vi "Initialize All DI Channels and TaskRefs.vi"(0 "DAQ":refnum<class "DAQ.lvclass">, 3 "DI Settings[]":T1[](array[typedef]), 5 "DAQNode Dict":T2, 7 "DI Tasks":T3[](array[typedef]), 11 "error in":errorcluster, 14 "Simulate":bool) -> (4 "DAQ out":refnum<class "DAQ.lvclass">, 6 "DAQNode Dict out":T2, 8 "DAQmxTaskDI[]":refnum<k21>[](array[refnum]), 10 "DI TaskNames":string[](array[string]), 15 "error out":errorcluster)   [LabVIEW 2017, in "DAQ.lvclass"]
doc: "Developed by Kevin Thompson\nkevin@thompsonengineering.net\n\nCopyright 2015\nThompson Engineering, LLC"
uses:
  DAQ.lvclass
  DataTypes/TD DI Task--cluster.ctl
  DataTypes/TD DI Channel--cluster.ctl
  <vilib>/TELLC/Dynamic CVT API/TD Dynamic CVT DVR--ref.ctl
  DataTypes/TD DI Instrument Settings--cluster.ctl
  DAQ.lvclass/DAQ.ctl
  Accessors/Set DI IONames.vi
  Accessors/Set DI SchemNames.vi
  Accessors/Set DI Settings.vi
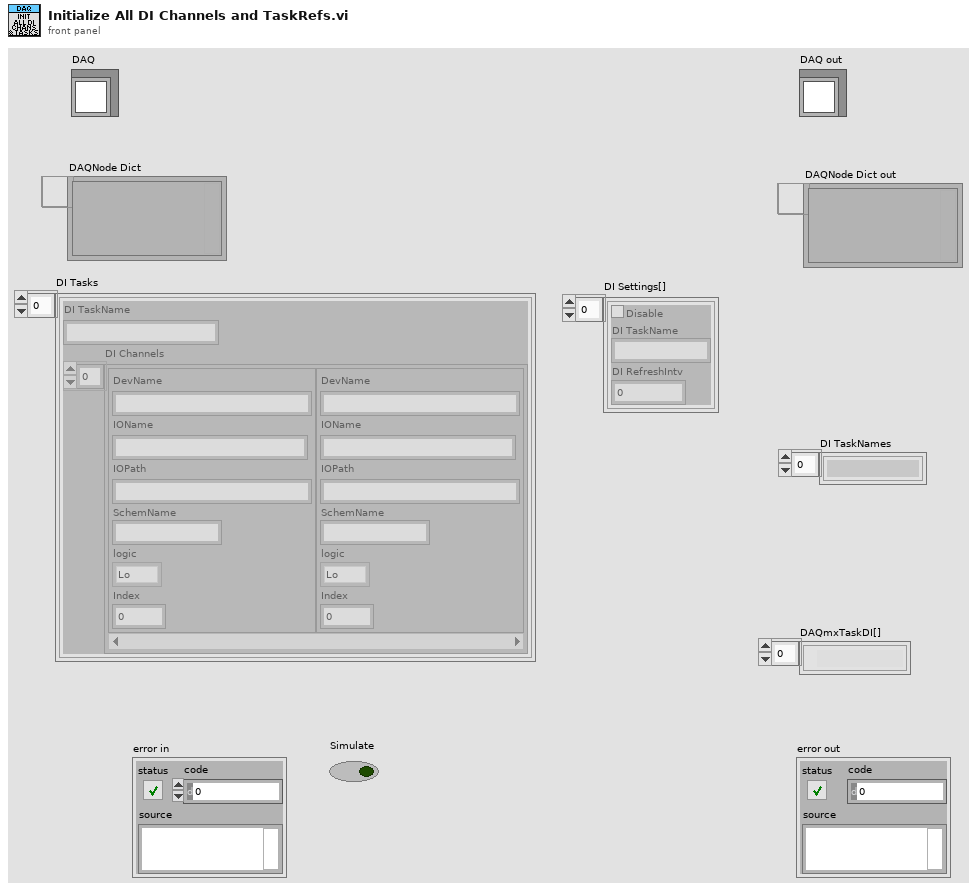
[diagram p1: front panel]
types:
  T1 = typedef "DAQ.lvclass/TD DI Instrument Settings--cluster.ctl" = cluster{"Disable":bool, "DI TaskName":string, "DI RefreshIntv":i32}
  T2 = typedef "TD Dynamic CVT DVR--ref.ctl" = refnum<data-value>
  T3 = typedef "DAQ.lvclass/TD DI Task--cluster.ctl" = cluster{"DI TaskName":string, "DI Channels":T4[]}
  T4 = typedef "DAQ.lvclass/TD DI Channel--cluster.ctl" = cluster{"DevName":string, "IOName":string, "IOPath":string, "SchemName":string, "logic":enum16{"Lo", "Hi"}, "Index":i32}
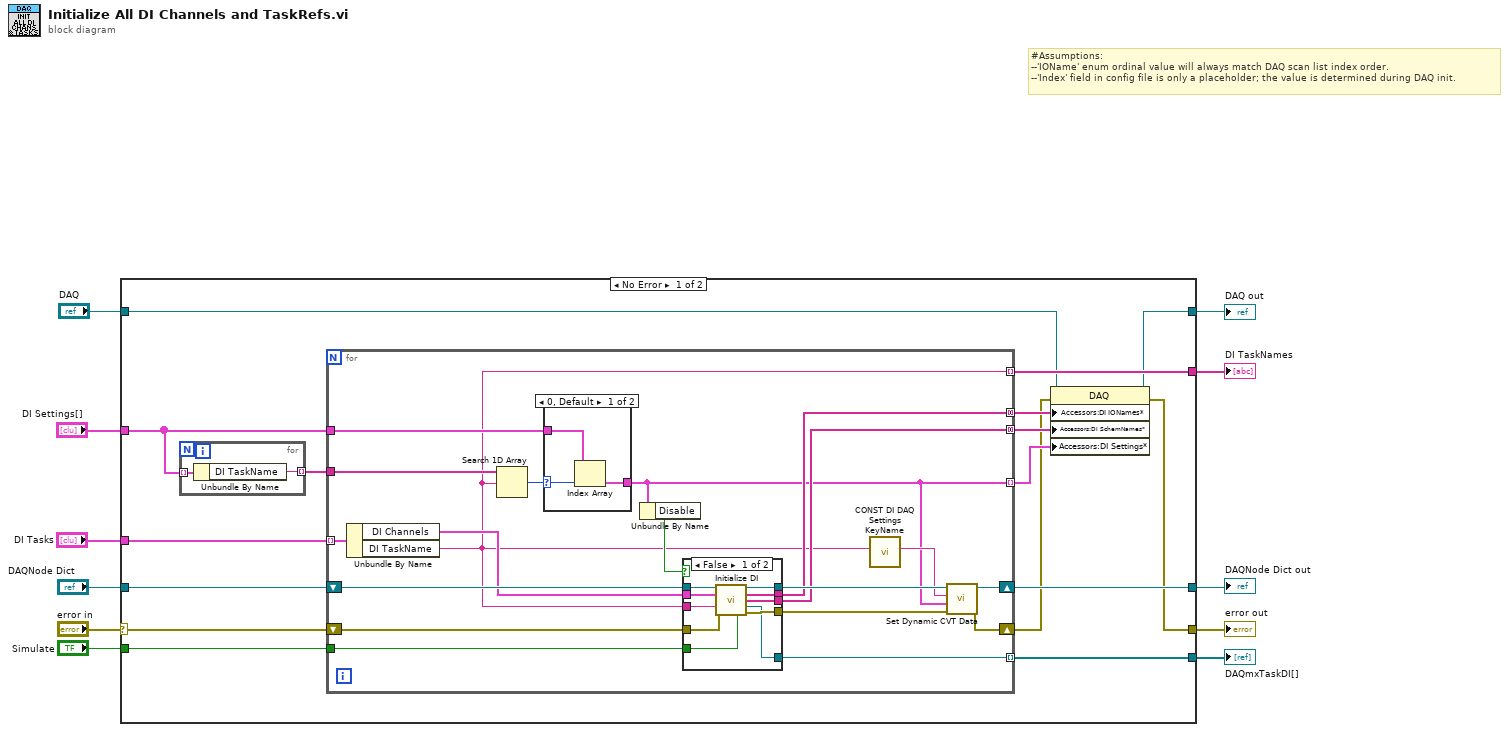
[diagram p0: block diagram]
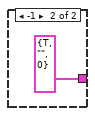
[diagram p3: hidden frame]
diagram:
  # "#Assumptions:\n--'IOName' enum ordinal value will always match DAQ scan list index order.\n--'Index' field in config file is only a placeholder; the value is determined during DAQ init."
  n1 = case shown="No Error" "error in" {
    selector: "error in" -> [w25 w67]
    tunnel: "DI Tasks" -> [w22 _]
    tunnel: "DAQNode Dict" -> [w27 w66]
    tunnel: [w12 w67] -> w9
    tunnel: [w24 w66] -> w4
    tunnel: "Simulate" -> [w26 _]
    tunnel: [w23 _] -> w6
    tunnel: "DI Settings[]" -> [w20 _]
    tunnel: [w19 _] -> w3
    tunnel: [w15 w65] -> w1
    tunnel: "DAQ" -> [w16 w65]
    frame No Error {
      n2 = for {
        tunnel: [w64] -> w21 mode=indexing
        tunnel: w20 -> [w63] mode=indexing
        n3 = Unbundle By Name(w63) -> ("DI TaskName"=w64:string)
      }
      n4 = for {
        tunnel: w26 -> [w34]
        tunnel: [w40] -> w23 mode=indexing
        shift-right: [w43] -> w24
        shift-left: w27 -> [w46]
        shift-right: [w44] -> w13
        shift-left: w25 -> [w45]
        tunnel: w22 -> [w39] mode=indexing
        tunnel: w21 -> [w37]
        tunnel: w20 -> [w35]
        tunnel: [w31] -> w18 mode=concatenating
        tunnel: [w30] -> w17 mode=concatenating
        tunnel: [w29] -> w19 mode=indexing
        tunnel: [w28] -> w14 mode=indexing
        n5 = Unbundle By Name(w39) -> ("DI Channels"=w38:T4[], "DI TaskName"=w29:string)
        n6 = Search 1D Array(1D array=w37, element=w29) -> (index of element=w36:i32)  [unwired: 1 in]
        n7 = case shown="0, Default" w36 {
          selector: w36 -> [w60 _]
          tunnel: [w61 T1 {"Disable"=TRUE, "DI TaskName"="", "DI RefreshIntv"=0} ("DI Settings")] -> w28
          tunnel: w35 -> [w59 _]
          frame 0, Default {
            n8 = Index Array(array=w59, index=w60) -> (element=w61:T1)
          }
          frame -1 {
          }
        }
        n9 = Unbundle By Name(w28) -> ("Disable"=w33:bool)
        n10 = case shown="False" w33 {
          tunnel: w46 -> [w56 w58]
          tunnel: w45 -> [w55 w57]
          tunnel: [w54 w58] -> w42
          tunnel: [w53 w57] -> w41
          tunnel: [w52 _] -> w40
          tunnel: w38 -> [w51 _]
          tunnel: w29 -> [w50 _]
          tunnel: w34 -> [w49 _]
          tunnel: [w48 _] -> w31
          tunnel: [w47 _] -> w30
          frame False {
            n11 = call "Initialize DI.vi"("DAQNode Dict"=w56, "DI Channels"=w51, "DI TaskName"=w50, "error in"=w55, "Simulate"=w49) -> ("DAQNode Dict out"=w54:T2, "DI IONames"=w48:string[], "DI SchemNames"=w47:string[], "DAQmx Task DI"=w52:refnum<k21>, "error out"=w53:errorcluster)  [unwired: 6 in]
          }
          frame True {
          }
        }
        n12 = call "CONST DI DAQ Settings KeyName.vi"("DI TaskName"=w29) -> ("DI DAQ Settings (KeyName)"=w32:string)  [unwired: 10 in]
        n13 = call <vilib>:"Set Dynamic CVT Data.vi"("error in (no error)"=w41, "value"=w28, "DataName"=w32, "dCVT DVR"=w42) -> ("error out"=w44:errorcluster, "dCVT DVR out"=w43:T2)  [unwired: 5 in, 1 out]
      }
      n14 = property class="DAQ"(reference=w16, error in=w13, "Accessors:DI IONames*"=w18, "Accessors:DI SchemNames*"=w17, "Accessors:DI Settings*"=w14) -> (reference out=w15:refnum<class "DAQ.lvclass">, error out=w12:errorcluster)
    }
    frame Error {
    }
  }
  "error out" <- w9
  "DAQNode Dict out" <- w4
  "DAQmxTaskDI[]" <- w6
  "DAQ out" <- w1
  "DI TaskNames" <- w3
